vi "Read Display Image.lvclass.vi"(8 "error in (no error)":errorcluster, 11 "Application in":refnum<class "Application.lvclass">) -> (0 "error out":errorcluster, 2 "Display Image.lvclass":refnum<class "Display Image.lvclass">, 3 "Application out":refnum<class "Application.lvclass">)   [LabVIEW 2018, in "Application.lvclass"]
uses:
  Application.lvclass
  Display Image/Display Image.lvclass
  Application.lvclass/Application.ctl
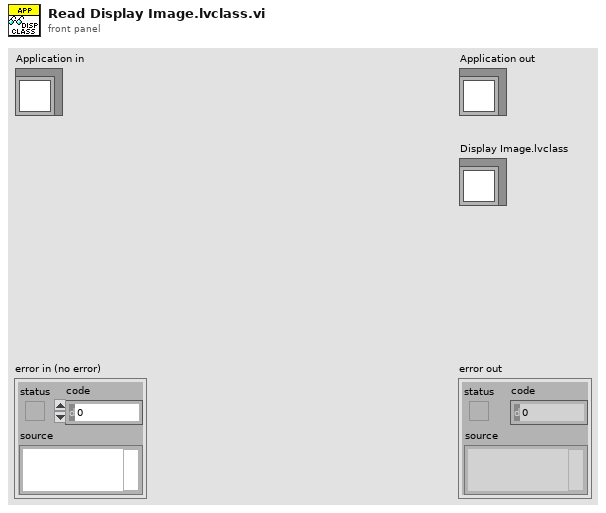
[diagram p1: front panel]
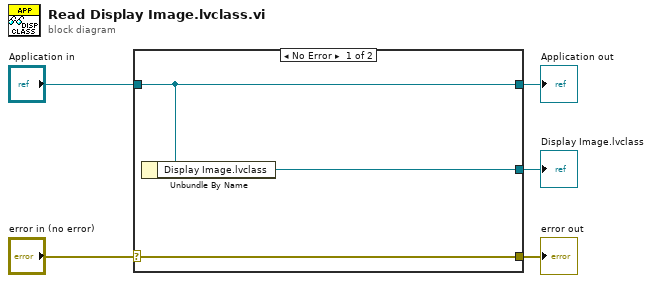
[diagram p0: block diagram]
diagram:
  n1 = case shown="No Error" "error in (no error)" {
    selector: "error in (no error)" -> [w8 w9]
    tunnel: [w8 w9] -> w4
    tunnel: [w7 w10] -> w2
    tunnel: "Application in" -> [w7 w10]
    tunnel: [w6 _] -> w1
    frame No Error {
      n2 = Unbundle By Name(w7) -> ("Display Image.lvclass"=w6:refnum<class "Display Image.lvclass">)
    }
    frame Error {
    }
  }
  "error out" <- w4
  "Application out" <- w2
  "Display Image.lvclass" <- w1
